vi "Lift To Inch.vi"(7 "Speed":dbl=1.0, 11 "Inches to move":dbl=10.016447368421053) -> (2 "Done":bool=TRUE)   [LabVIEW 2014]
uses:
  Begin/Global Variables.vi
  <vilib>/Rock Robotics/Network Tables/SD Write Boolean.vi
  Begin/Global RefNums.vi
  <vilib>/Rock Robotics/Network Tables/SD Write Number.vi
panel:
  in  "down speed":dbl=0.75
  in  "lower limit":dbl=0.5
  in  "normalize":dbl=0.834
  in  "inches slowed":dbl=10.0
  in  "Dec Constant":dbl=-2.0
  in  "slave offset":dbl=1800.0
  in  "right PID gains":T1={"proportional gain (Kc)"=0.0006, "integral time (Ti, min)"=0.0, "derivative time (Td, min)"=0.0003} {"derivative time (Td, min)" format="%.4f"; "integral time (Ti, min)" format="%.6f"; "proportional gain (Kc)" format="%.5f"}
  in  "left PID gains":T2={"proportional gain (Kc)"=0.002, "integral time (Ti, min)"=0.0, "derivative time (Td, min)"=0.0005} {"derivative time (Td, min)" format="%.10f"; "proportional gain (Kc)" format="%.5f"}
  in  "Output Range":cluster{"output high":dbl, "output low":dbl}={"output high"=0.5, "output low"=-0.5} {"output low" format="%.2f"; "output high" format="%.2f"}
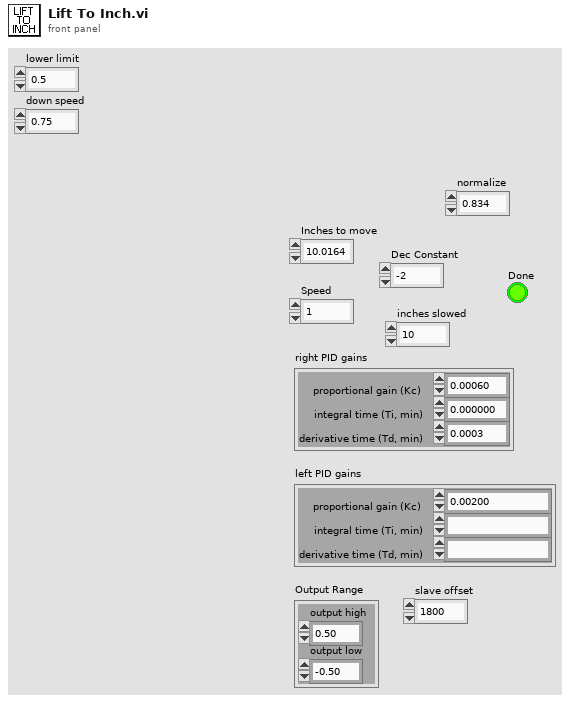
[diagram p1: front panel]
types:
  T1 = cluster{"proportional gain (Kc)":dbl, "integral time (Ti, min)":dbl, "derivative time (Td, min)":dbl}
  T2 = cluster{"proportional gain (Kc)":dbl, "integral time (Ti, min)":fxp<+/-,64,32>, "derivative time (Td, min)":dbl}
  T3 = typedef "WPI_EncoderDevRef.ctl" = cluster{"DevStatus":errorcluster, "EncoderIndex":T4, "CounterIndex":T5, "DistancePerCount":dbl, "Decoding Type":T6}
  T4 = typedef "FPGA_EncoderIdx.ctl" = enum8{"Enc 0", "Enc 1", "Enc 2", "Enc 3", "Enc 4", "Enc 5", "Enc 6", "Enc 7", "Invalid"}
  T5 = typedef "FPGA_CounterCtrSystemIndex.ctl" = enum8{"Ctr 0", "Ctr 1", "Ctr 2", "Ctr 3", "Ctr 4", "Ctr 5", "Ctr 6", "Ctr 7", "Invalid"}
  T6 = typedef "WPI_EncoderType.ctl" = enum16{"1x", "2x", "4x"}
  T7 = typedef "WPI_MotorControlDeviceRef.ctl" = cluster{"DeviceStatus":errorcluster, "Type":T8, "PWM":cluster{"Controller":T9, "PWM Channel":T10, "DeadBand":T11}, "CAN":cluster{"Device Number":u8, "Control Mode":T12, "Semaphore":T13, "Max Vout":dbl, "TalonSRX Control Mode":T14}, "Invert":bool, "TransformRef":T15, "InvTransformRef":T15}
  T8 = typedef "WPI_MotorControlType.ctl" = enum16{"PWM", "CAN", "CANTalonSRX"}
  T9 = typedef "FPGA_TypedefDigitalModule.ctl" = enum16{"Controller 1"}
  T10 = typedef "FPGA_DIOPWMChannel.ctl" = enum8{"PWM 0", "PWM 1", "PWM 2", "PWM 3", "PWM 4", "PWM 5", "PWM 6", "PWM 7", "PWM 8", "PWM 9", "PWM MXP 0", "PWM MXP 1", "PWM MXP 2", "PWM MXP 3", "PWM MXP 4", "PWM MXP 5", "PWM MXP 6", "PWM MXP 7", "PWM MXP 8", "PWM MXP 9", "Invalid"}
  T11 = typedef "WPI_PWMDeadband.ctl" = cluster{"Name":string, "maxPositivePwm":i32, "minPositivePwm":i32, "centerPwm":i32, "maxNegativePwm":i32, "minNegativePwm":i32, "angularRange":u16}
  T12 = typedef "WPI_CANJaguar_ControlMode.ctl" = enum8{"Percent VBus", "Current", "Speed", "Position", "Voltage"}
  T13 = typedef "Semaphore RefNum" = refnum<k1>
  T14 = typedef "WPI_CANTalonSRX_APIControlMode.ctl" = enum8{"Percent VBus", "Speed", "Position", "Slave", "Unchanged / Invalid"}
  T15 = typedef "WPI_PWMTransform_ConPane.ctl" = refnum<vi>
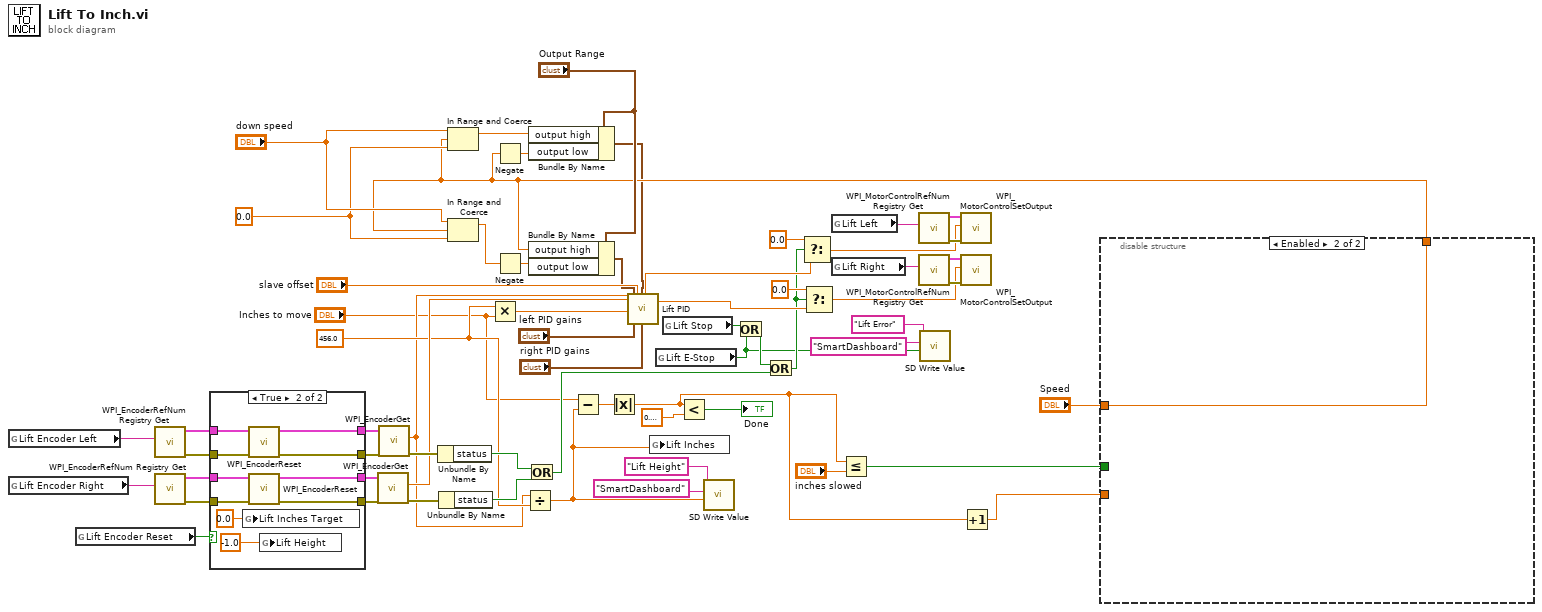
[diagram p0: block diagram]
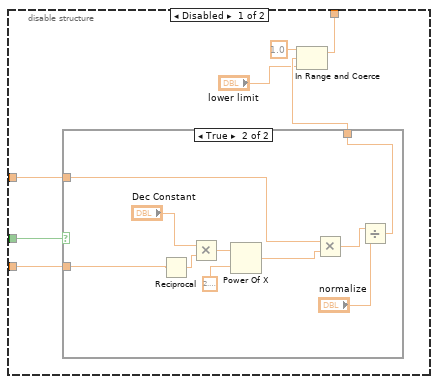
[diagram p2: hidden frame]
diagram:
  w7 = 0.0 ("lower limit")
  w18 = 456.0 ("y")
  n1 = global read "Global RefNums.vi" "Lift Encoder Left"() -> (w28:string)
  n2 = global read "Global RefNums.vi" "Lift Encoder Right"() -> (w27:string)
  n3 = global read "Global Variables.vi" "Lift Encoder Reset"() -> (w17:bool)
  n4 = call <vilib>:"WPI_EncoderRefNum Registry Get.vi"("refnum name"=w28) -> ("error out"=w58:errorcluster, "EncoderDevRef"=w57:T3)  [unwired: 9 in]
  n5 = call <vilib>:"WPI_EncoderRefNum Registry Get.vi"("refnum name"=w27) -> ("error out"=w55:errorcluster, "EncoderDevRef"=w56:T3)  [unwired: 9 in]
  n6 = case shown="True" w17 {
    tunnel: w55 -> [w64 w77]
    tunnel: w56 -> [w65 w76]
    tunnel: w58 -> [w66 w74]
    tunnel: w57 -> [w67 w75]
    tunnel: [w67 w73] -> w60
    tunnel: [w65 w72] -> w61
    tunnel: [w64 w71] -> w62
    tunnel: [w66 w70] -> w63
    frame False {
    }
    frame True {
      n7 = global write "Global Variables.vi" "Lift Inches Target"(0.0 ("Lift Inches Target")) -> ()
      n8 = call <vilib>:"WPI_EncoderReset.vi"("error in (no error)"=w74, "EncoderDevRef"=w75) -> ("error out"=w70:errorcluster, "EncoderDevRef"=w73:T3)  [unwired: 8 in]
      n9 = call <vilib>:"WPI_EncoderReset.vi"("error in (no error)"=w77, "EncoderDevRef"=w76) -> ("error out"=w71:errorcluster, "EncoderDevRef"=w72:T3)  [unwired: 8 in]
      n10 = global write "Global Variables.vi" "Lift Height"(-1.0 ("Lift Inches Target")) -> ()
    }
  }
  n11 = call <vilib>:"WPI_EncoderGet.vi"("error in (no error)"=w62, "EncoderDevRef"=w61) -> ("error out"=w34:errorcluster, "Distance"=w25:dbl)  [unwired: 4 in, 4 out]
  n12 = call <vilib>:"WPI_EncoderGet.vi"("error in (no error)"=w63, "EncoderDevRef"=w60) -> ("error out"=w37:errorcluster, "Distance"=w16:dbl)  [unwired: 4 in, 4 out]
  n13 = Unbundle By Name(w37) -> ("status"=w35:bool)
  n14 = Unbundle By Name(w34) -> ("status"=w33:bool)
  n15 = Multiply(x=w18, y="Inches to move") -> (x*y=w47:dbl)
  n16 = Divide(x=w16, y=w18) -> (x/y=w22:dbl)
  n17 = Or(x=w35, y=w33) -> (x .or. y?=w32:bool)
  n18 = Subtract(x="Inches to move", y=w22) -> (x-y=w46:dbl)
  n19 = Absolute Value(x=w46) -> (abs(x)=w12:dbl)
  n20 = global write "Global Variables.vi" "Lift Inches"(w22) -> ()
  n21 = global read "Global Variables.vi" "Lift E-Stop"() -> (w19:bool)
  n22 = global read "Global Variables.vi" "Lift Stop"() -> (w26:bool)
  n23 = Less?(x=w12, y=0.20000000000000004) -> (x < y?=→"Done":bool)
  n24 = call-poly <vilib>:"SD Write Value.vi"("Numeric"=w22, "Table Prefix"="SmartDashboard", "Name"="Lift Height") -> ()  [unwired: 7 in, 2 out]
  n25 = Or(x=w26, y=w19) -> (x .or. y?=w31:bool)
  n26 = Or(x=w31, y=w32) -> (x .or. y?=w36:bool)
  n27 = global read "Global RefNums.vi" "Lift Left"() -> (w30:string)
  n28 = global read "Global RefNums.vi" "Lift Right"() -> (w29:string)
  n29 = Less Or Equal?(x=w12, y="inches slowed") -> (x <= y?=w14:bool)
  n30 = call <vilib>:"WPI_MotorControlRefNum Registry Get.vi"("refnum name"=w30) -> ("error out"=w52:errorcluster, "MotorControlDevRef"=w51:T7)  [unwired: 9 in]
  n31 = call <vilib>:"WPI_MotorControlRefNum Registry Get.vi"("refnum name"=w29) -> ("error out"=w49:errorcluster, "MotorControlDevRef"=w50:T7)  [unwired: 9 in]
  n32 = call-poly <vilib>:"SD Write Value.vi"("Boolean"=w19, "Table Prefix"="SmartDashboard", "Name"="Lift Error") -> ()  [unwired: 7 in, 2 out]
  n33 = Increment(x=w12) -> (x+1=w11:dbl)
  n34 = disable-structure shown="Enabled" {
    disable-tunnel: w14 -> [w84 _]
    disable-tunnel: "Speed" -> [w83 w96]
    disable-tunnel: w11 -> [w82 _]
    disable-tunnel: [w78 w96] -> w4
    frame Disabled {
      n35 = case shown="True" w84 {
        tunnel: w83 -> [w85 w92]
        tunnel: [w85 w87] -> w81
        tunnel: w82 -> [_ w90]
        frame False {
        }
        frame True {
          n36 = Reciprocal(x=w90) -> (1/x=w89:dbl)
          n37 = Multiply(x="Dec Constant", y=w89) -> (x*y=w93:dbl)
          n38 = Power Of X(1:2.718281828459045, 2:w93) -> (0:w91:dbl)
          n39 = Multiply(x=w92, y=w91) -> (x*y=w88:dbl)
          n40 = Divide(x=w88, y="normalize") -> (x/y=w87:dbl)
        }
      }
      n41 = In Range and Coerce(upper limit=1.0, x=w81, lower limit="lower limit") -> (coerced(x)=w78:dbl)  [unwired: 1 out]
    }
    frame Enabled {
    }
  }
  n42 = In Range and Coerce(upper limit="down speed", x=w4, lower limit=w7) -> (coerced(x)=w3:dbl)  [unwired: 1 out]
  n43 = In Range and Coerce(upper limit="down speed", x=w4, lower limit=w7) -> (coerced(x)=w9:dbl)  [unwired: 1 out]
  n44 = Negate(x=w4) -> (-x=w5:dbl)
  n45 = Negate(x=w9) -> (-x=w48:dbl)
  n46 = Bundle By Name(cluster="Output Range", "output high"=w3, "output low"=w5) -> (w2:cluster{"output high":dbl, "output low":dbl})
  n47 = Bundle By Name(cluster="Output Range", "output high"=w4, "output low"=w48) -> (w1:cluster{"output high":dbl, "output low":dbl})
  n48 = call "Lift PID.vi"("left encoder"=w16, "right encoder"=w25, "move to distance"=w47, "left output range"=w1, "left PID gains"="left PID gains", "slave offset"="slave offset", "right output range"=w2, "right PID gains"="right PID gains") -> ("lift motor left"=w38:dbl, "lift motor right"=w39:dbl)  [unwired: 18 in]
  n49 = Select(t=0.0, s=w36, f=w38) -> (s? t:f=w41:dbl)
  n50 = Select(t=0.0, s=w36, f=w39) -> (s? t:f=w40:dbl)
  n51 = call <vilib>:"WPI_MotorControlSetOutput.vi"("error in (no error)"=w52, "Output"=w41, "MotorControlDevRef"=w51) -> ()  [unwired: 6 in, 3 out]
  n52 = call <vilib>:"WPI_MotorControlSetOutput.vi"("error in (no error)"=w49, "Output"=w40, "MotorControlDevRef"=w50) -> ()  [unwired: 6 in, 3 out]
